vi "ListControlNames.vi"(8 "error in (no error)":errorcluster, 10 "NameSpace (empty)":string, 11 "FlattenControls[]":refnum<vi>[](array[refnum])) -> (0 "error out":errorcluster, 3 "Array":string[](array[string]))   [LabVIEW 2021]
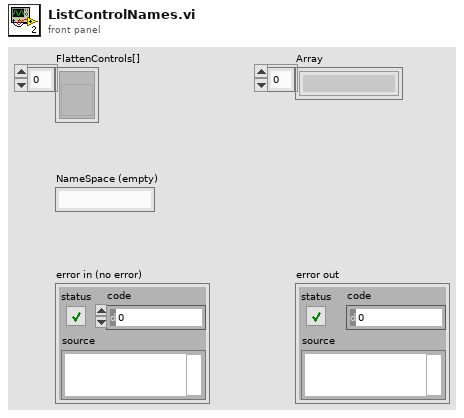
[diagram p1: front panel]
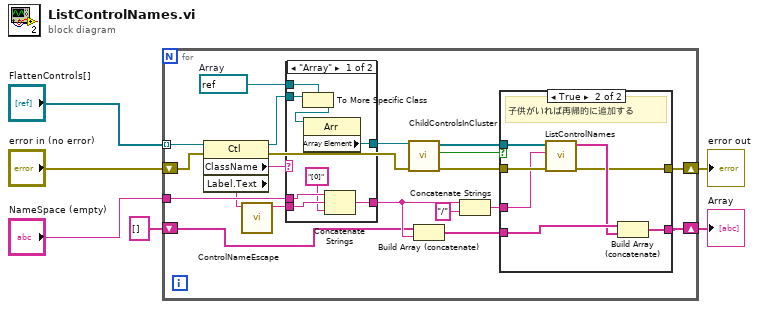
[diagram p0: block diagram]
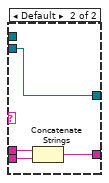
[diagram p2: hidden frame]
diagram:
  n1 = for {
    tunnel: "FlattenControls[]" -> [w26] mode=indexing
    shift-right: [w24] -> w4
    shift-left: string[] [] -> [w12]
    shift-right: [w18] -> w2
    shift-left: "error in (no error)" -> [w21]
    tunnel: "NameSpace (empty)" -> [w17]
    w8 = refnum<vi> refnum  # Array
    n2 = property class="Ctl"(reference=w26, error in=w21) -> (reference out=w9:refnum<vi>, error out=w20:errorcluster, "ClassName"=w10:string, "Label.Text"=w11:string)
    n3 = call "ControlNameEscape.vi"("label"=w11) -> ("escaped string"=w13:string)  [unwired: 10 in]
    n4 = case shown="\"Array\"" w10 {
      tunnel: w17 -> [w34 w38]
      tunnel: [w33 w37] -> w16
      tunnel: w13 -> [w28 w36]
      tunnel: w9 -> [w31 w35]
      tunnel: w8 -> [w30 _]
      tunnel: [w29 w35] -> w7
      frame "Array" {
        n5 = To More Specific Class(target class=w30, reference=w31) -> (specific class reference=w32:refnum<vi>)  [unwired: 1 in, 1 out]
        n6 = property class="Arr"(reference=w32) -> ("Array Element"=w29:refnum<vi>)  [unwired: 1 in, 2 out]
        n7 = Concatenate Strings(w34, w28, "[0]" ("string")) -> (w33:string)
      }
      frame Default {
        n8 = Concatenate Strings(w38, w36) -> (w37:string)
      }
    }
    n9 = call "ChildControlsInCluster.vi"("error in (no error)"=w20, "Control in"=w7) -> ("error out"=w19:errorcluster, "IsCluster"=w23:bool, "Controls[]"=w22:refnum<vi>[])  [unwired: 7 in]
    n10 = Build Array (concatenate)(w12, w16) -> (w25:string[])
    n11 = Concatenate Strings(w16, "/" ("string")) -> (w14:string)
    n12 = case shown="True" w23 {
      tunnel: w25 -> [w40 w46]
      tunnel: [w40 w44] -> w24
      tunnel: w22 -> [_ w47]
      tunnel: w19 -> [w39 w43]
      tunnel: [w39 w42] -> w18
      tunnel: w14 -> [_ w41]
      frame False {
      }
      frame True {
        # "子供がいれば再帰的に追加する"
        n13 = call "ListControlNames.vi"("error in (no error)"=w43, "NameSpace (empty)"=w41, "FlattenControls[]"=w47) -> ("error out"=w42:errorcluster, "Array"=w45:string[])  [unwired: 7 in]
        n14 = Build Array (concatenate)(w46, w45) -> (w44:string[])
      }
    }
  }
  "Array" <- w4
  "error out" <- w2
